vi "Write PPSTime.vi"(8 "error in (no error)":errorcluster, 10 "PPSTime":dbl, 11 "SyncPluginBase in":refnum<class "SyncPluginBase.lvclass">) -> (0 "error out":errorcluster, 3 "SyncPluginBase out":refnum<class "SyncPluginBase.lvclass">)   [LabVIEW 2014, in "SyncPlugins.lvlib" / "SyncPluginBase.lvclass"]
uses:
  SyncPluginBase.lvclass
  SyncPluginBase.lvclass/SyncPluginBase.ctl
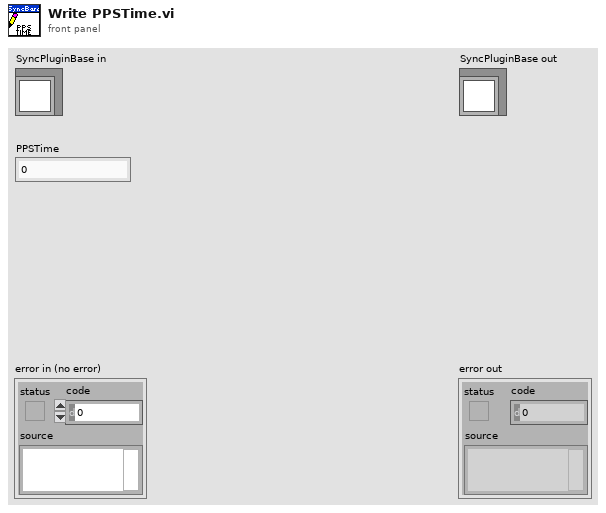
[diagram p1: front panel]
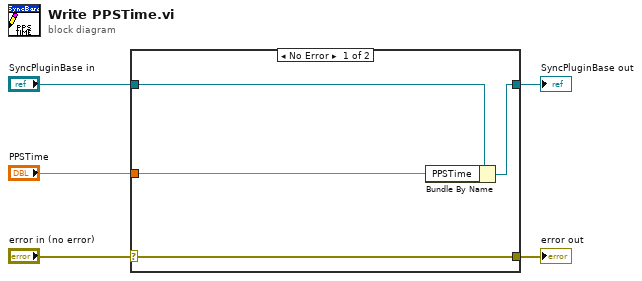
[diagram p0: block diagram]
diagram:
  n1 = case shown="No Error" "error in (no error)" {
    selector: "error in (no error)" -> [w9 w10]
    tunnel: [w9 w10] -> w4
    tunnel: [w7 w11] -> w2
    tunnel: "SyncPluginBase in" -> [w8 w11]
    tunnel: "PPSTime" -> [w6 _]
    frame No Error {
      n2 = Bundle By Name(cluster=w8, "PPSTime"=w6) -> (w7:refnum<class "SyncPluginBase.lvclass">)
    }
    frame Error {
    }
  }
  "error out" <- w4
  "SyncPluginBase out" <- w2
